vi "Main.vi"() -> ()   [LabVIEW 2024]
uses:
  Circulo_class/Circulo.lvclass
  C:/GitClones/LabVIEW-GYM/Sesiones/Sesiones/Sesion [10] 30 Junio 2025/Ejercicio UML/FiguraGeometrica_interface/FiguraGeometrica.lvclass
  Rectangulo_class/Rectangulo.lvclass
  Triangulo.lvclass
  Rectangulo_class/Rectangulo.lvclass/Rectangulo.ctl
  Triangulo.lvclass/Triangulo.ctl
  Circulo_class/Circulo.lvclass/Circulo.ctl
  Write Altura.vi
  Write Base.vi
  Rectangulo_class/Write Altura.vi
  Rectangulo_class/Write Base.vi
  Circulo_class/Write Radio.vi
  FiguraGeometrica_interface/FiguraGeometrica.lvclass
panel:
  out "Array":dbl[](array[numeric])
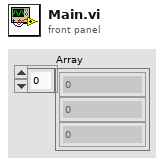
[diagram p1: front panel]
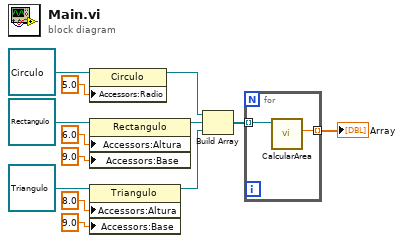
[diagram p0: block diagram]
diagram:
  n1 = property class="Circulo"(reference=refnum<class "Circulo.lvclass"> refnum ("Circulo"), "Accessors:Radio"=5.0 ("Radio")) -> (reference out=w5:refnum<class "Circulo.lvclass">)  [unwired: 1 in, 1 out]
  n2 = property class="Rectangulo"(reference=refnum<class "Rectangulo.lvclass"> refnum ("Rectangulo"), "Accessors:Altura"=6.0 ("Altura"), "Accessors:Base"=9.0 ("Base")) -> (reference out=w4:refnum<class "Rectangulo.lvclass">)  [unwired: 1 in, 1 out]
  n3 = property class="Triangulo"(reference=refnum<class "Triangulo.lvclass"> refnum ("Triangulo"), "Accessors:Altura"=8.0 ("Altura"), "Accessors:Base"=9.0 ("Base")) -> (reference out=w3:refnum<class "Triangulo.lvclass">)  [unwired: 1 in, 1 out]
  n4 = Build Array(w5, w4, w3) -> (w2:refnum<class "FiguraGeometrica.lvclass">[])
  n5 = for {
    tunnel: w2 -> [w15] mode=indexing
    tunnel: [w14] -> w1 mode=indexing
    n6 = call-dynamic "CalcularArea.vi"("object in"=w15) -> ("Area"=w14:dbl)  [unwired: 8 in, 2 out]
  }
  "Array" <- w1
